vi "SMU_1 CH_ Guardian Meas.vi"(6 "script name":string="IDD", 7 "Meas_A_Level":dbl=0.01, 8 "error in (no error)":errorcluster, 9 "Publishable IDs":string[](array[string])=["IDD_LowPower", "IDD_DVC_Cmin", "IDD_DVC_Cmax"], 10 "Pin":string[](array[string])=["VDD"], 11 "Semiconductor Module Context":T1) -> (0 "error out":errorcluster)   [LabVIEW 2013]
uses:
  <vilib>/NI_TestStand_SemiconductorModule/NI_TestStand_Semiconductor_Module.lvlibp/PinMap/General/SemiconductorModuleContext.ctl
  <instrlib>/niHSDIO/niHSDIO.llb/niHSDIO_ctl Trigger Script - trigID Values (Ring).ctl
  <vilib>/NI_TestStand_SemiconductorModule/NI_TestStand_Semiconductor_Module.lvlibp
panel:
  out "R Array":dbl[][](array[numeric])
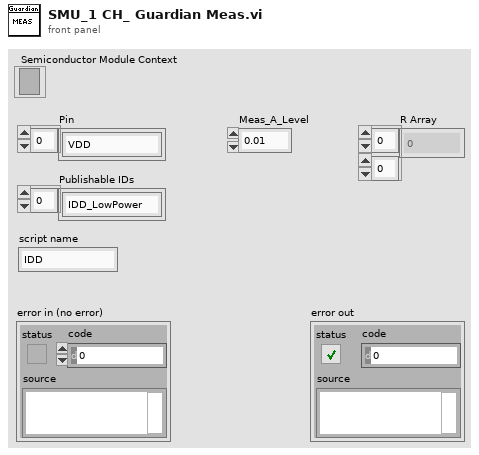
[diagram p1: front panel]
types:
  T1 = typedef "NI_TestStand_Semiconductor_Module.lvlibp/SemiconductorModuleContext.ctl" = refnum<k7>
  T2 = typedef "niHSDIO_ctl Trigger Script - trigID Values (Ring).ctl" = string
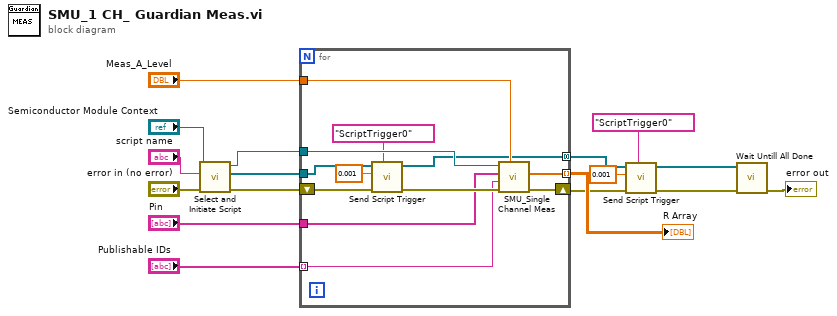
[diagram p0: block diagram]
diagram:
  n1 = call "Select and Initiate Script.vi"("error in (no error)"="error in (no error)", "script name"="script name", "Semiconductor Module Context"="Semiconductor Module Context") -> ("error out"=w14:errorcluster, "HSDIO GEN Sessions Out"=w10:refnum<k15>[], "Semiconductor Module Context Out"=w11:T1)  [unwired: 6 in]
  n2 = for {
    tunnel: "Publishable IDs" -> [w22] mode=indexing
    tunnel: "Pin" -> [w23]
    tunnel: w11 -> [w29]
    tunnel: w10 -> [w28]
    tunnel: "Meas_A_Level" -> [w24]
    shift-right: [w21] -> w4
    shift-left: w14 -> [w26]
    tunnel: [w20] -> w6 mode=concatenating
    tunnel: [w19] -> w8 mode=indexing
    n3 = call "Send Script Trigger.vi"("trigger id (script trigger 0)"=T2 "ScriptTrigger0", "error in (no error)"=w26, "Delay Time (s)"=0.001, "HSDIO Sessions In"=w28) -> ("error out"=w25:errorcluster, "HSDIO Sessions Out"=w20:refnum<k15>[])  [unwired: 6 in]
    n4 = call "SMU_Single Channel Meas.vi"("Meas_A_Level"=w24, "error in (no error)"=w25, "Published Data Id"=w22, "Pins"=w23, "Semiconductor Module Context"=w29) -> ("error Out"=w21:errorcluster, "R Array"=w19:dbl[])  [unwired: 4 in, 1 out]
  }
  "R Array" <- w8
  n5 = call "Send Script Trigger.vi"("trigger id (script trigger 0)"=T2 "ScriptTrigger0", "error in (no error)"=w4, "Delay Time (s)"=0.001, "HSDIO Sessions In"=w6) -> ("error out"=w3:errorcluster, "HSDIO Sessions Out"=w5:refnum<k15>[])  [unwired: 6 in]
  n6 = call "Wait Untill All Done.vi"("error in (no error)"=w3, "HSDIO Sessions In"=w5) -> ("error out"=→"error out":errorcluster)  [unwired: 8 in, 1 out]
